vi "TestBuild.vi"   [LabVIEW 2020]
uses:
  ECU_Diagnose/ECU_Diagnose.lvlibp
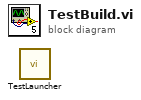
[diagram p0: block diagram]
diagram:
  n1 = call "TestLauncher.vi"() -> ()  [unwired: 20 in]
